vi "Initialize Sessions - 1Sess.vi"(6 "initialize and close session behavior":T1, 7 "option string":string, 8 "error in":errorcluster, 9 "reset":bool, 11 "session reservation in":refnum<class "Session Reservation.lvclass">) -> (0 "error out":errorcluster, 1 "channel list":string, 2 "session":refnum<k15>, 3 "session reservation out":refnum<class "Session Reservation.lvclass">)   [LabVIEW 2020, in "Plug-In SDK niDigital Sessions.lvlib"]
doc: "Create the NI-Digital driver session from the <b>session reservation in</b>. Returns an error if more than one NI-Digital session has been reserved. Use \"Create Session - NSess.vi\" for multiple sessions."
uses:
  Plug-In SDK niDigital Sessions.lvlib
  7f77feb2-d2b5-4acd-8f0f-f1b24b7d1641.vi
  Session Factory/Session Factory.lvclass
  Clients/Session Management V1/Session Reservation/Session Reservation.lvclass
  Clients/Session Management V1/Session Reservation/Initialize and Close Session Behavior.ctl
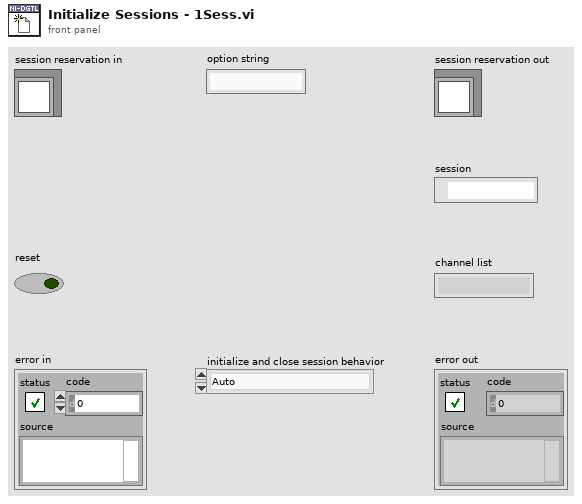
[diagram p1: front panel]
types:
  T1 = typedef "NI Session Management V1 Client.lvlib/Session Reservation.lvclass/Initialize and Close Session Behavior.ctl" = enum16{"Auto", "Initialize and Close", "Attach and Detach", "Initialize and Detach", "Attach and Close"}
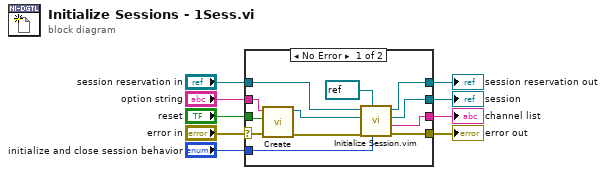
[diagram p0: block diagram]
diagram:
  n1 = case shown="No Error" "error in" {
    selector: "error in" -> [w16 w23]
    tunnel: [w20 w23] -> w8
    tunnel: [w21 w22] -> w6
    tunnel: "session reservation in" -> [w17 w22]
    tunnel: "option string" -> [w14 _]
    tunnel: "reset" -> [w15 _]
    tunnel: [w19 _] -> w3
    tunnel: [w18 _] -> w2
    tunnel: "initialize and close session behavior" -> [w10 _]
    frame No Error {
      n2 = call "Create.vi"("error in"=w16, "reset"=w15, "option string"=w14) -> ("error out"=w12:errorcluster, "session factory out"=w13:refnum<class "Session Factory.lvclass">)  [unwired: 7 in]
      n3 = call "Initialize Session.vim"("initialize and close session behavior"=w10, "session type"=refnum<k15> refnum ("instrument handle"), "error in"=w12, "session factory"=w13, "session reservation in"=w17) -> ("error out"=w20:errorcluster, "channel list"=w19:string, "session"=w18:refnum<k15>, "session reservation out"=w21:refnum<class "Session Reservation.lvclass">)  [unwired: 3 in]
    }
    frame Error {
    }
  }
  "error out" <- w8
  "session reservation out" <- w6
  "session" <- w2
  "channel list" <- w3
